vi "Array-Rectify.vi"(1 "Array":dbl[][](array[numeric])) -> (0 "Rectified Array":dbl[][](array[numeric]))   [LabVIEW 2020]
uses:
  <vilib>/Analysis/NI_AALPro.lvlib
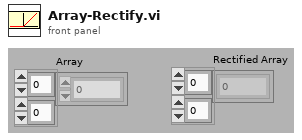
[diagram p1: front panel]
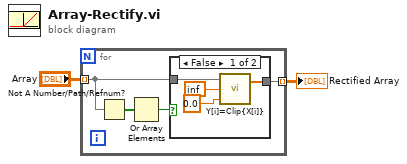
[diagram p0: block diagram]
diagram:
  n1 = for {
    tunnel: "Array" -> [w5] mode=indexing
    tunnel: [w6] -> w1 mode=indexing
    n2 = Not A Number/Path/Refnum?(number/path/refnum=w5) -> (NaN/Path/Refnum?=w4:bool[])
    n3 = Or Array Elements(Boolean array=w4) -> (logical OR=w3:bool)
    n4 = case shown="False" w3 {
      tunnel: [w8 w11] -> w6
      tunnel: w5 -> [w7 w11]
      frame False {
        n5 = call <vilib>:"Y[i]=Clip{X[i]}.vi"("lower limit"=0.0, "upper limit"=inf, "Input Array"=w7) -> ("Clipped Array"=w8:dbl[])  [unwired: 1 out]
      }
      frame True {
      }
    }
  }
  "Rectified Array" <- w1
